vi "Add Numeric Default Value Node.vi"(8 "error in":errorcluster, 9 "Default Value":string, 10 "Element in":refnum<k20>, 11 "Document in":refnum<k20>) -> (0 "error out":errorcluster, 2 "Element out":refnum<k20>, 3 "Document out":refnum<k20>)   [LabVIEW 2025]
uses:
  <resource>/objmgr/DOMUserDefRef.rc
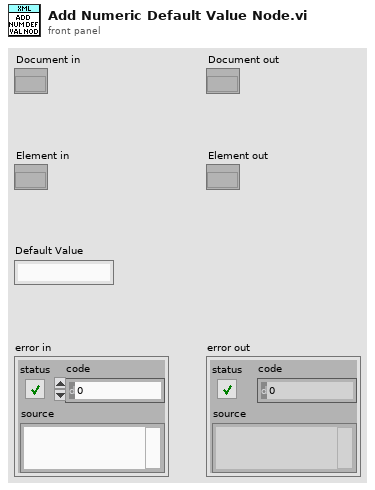
[diagram p1: front panel]
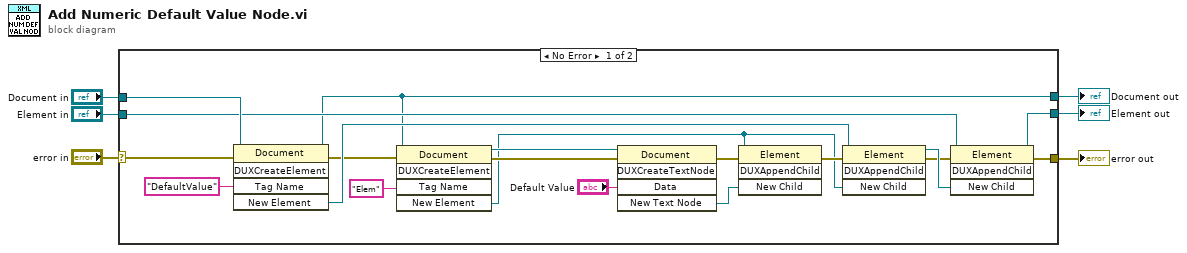
[diagram p0: block diagram]
diagram:
  n1 = case shown="No Error" "error in" {
    selector: "error in" -> [w7 w28]
    tunnel: "Document in" -> [w15 w26]
    tunnel: "Element in" -> [w14 w27]
    tunnel: [w10 w28] -> w4
    tunnel: [w9 w27] -> w3
    tunnel: [w8 w26] -> w2
    frame No Error {
      n2 = invoke class="Document" method="DUXCreateElement"(reference=w15, error in=w7, "Tag Name"="DefaultValue") -> (reference out=w8:refnum<k20>, error out=w12:errorcluster, "New Element"=w13:refnum<k20>)  [unwired: 2 in, 2 out]
      n3 = invoke class="Document" method="DUXCreateElement"(reference=w8, error in=w12, "Tag Name"="Elem") -> (reference out=w20:refnum<k20>, error out=w25:errorcluster, "New Element"=w17:refnum<k20>)  [unwired: 2 in, 2 out]
      n4 = invoke class="Document" method="DUXCreateTextNode"(reference=w20, error in=w25, "Data"="Default Value") -> (error out=w23:errorcluster, "New Text Node"=w19:refnum<k20>)  [unwired: 2 in, 3 out]
      n5 = invoke class="Element" method="DUXAppendChild"(reference=w17, error in=w23, "New Child"=w19) -> (error out=w24:errorcluster)  [unwired: 1 in, 3 out]
      n6 = invoke class="Element" method="DUXAppendChild"(reference=w13, error in=w24, "New Child"=w17) -> (reference out=w16:refnum<k20>, error out=w11:errorcluster)  [unwired: 1 in, 2 out]
      n7 = invoke class="Element" method="DUXAppendChild"(reference=w14, error in=w11, "New Child"=w16) -> (reference out=w9:refnum<k20>, error out=w10:errorcluster)  [unwired: 1 in, 2 out]
    }
    frame Error {
    }
  }
  "error out" <- w4
  "Element out" <- w3
  "Document out" <- w2
